vi "sv_Check for Midband Frequency Change.vi"(8 "error in (no error)":errorcluster, 10 "midband frequency setting":T1, 11 "reset filter (F)":bool) -> (0 "error out":errorcluster, 3 "parameter has changed":bool)   [LabVIEW 2017, in "SoundVib_Octave_2014 standard.lvlib"]
uses:
  <vilib>/addons/Sound and Vibration/svt_Octave/SoundVib_Octave_2014 standard.lvlib
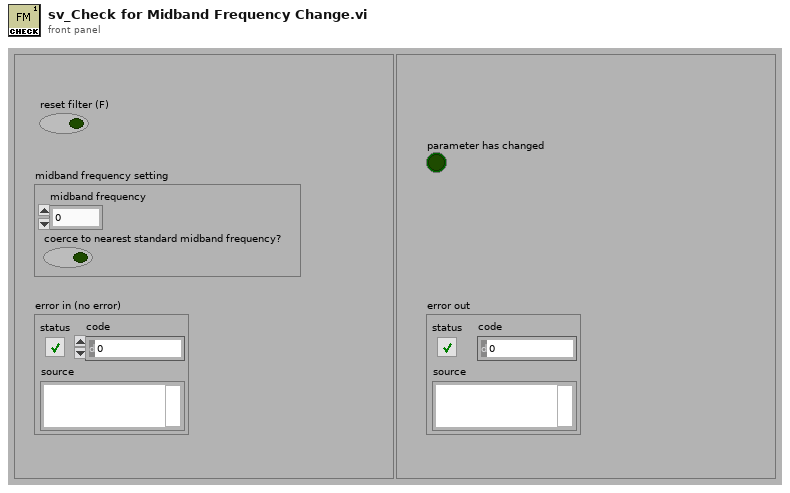
[diagram p1: front panel]
types:
  T1 = cluster{"midband frequency":dbl, "coerce to nearest standard midband frequency?":bool}
  T2 = cluster{"midband frequency":bool, "coerce to nearest standard midband frequency?":bool}
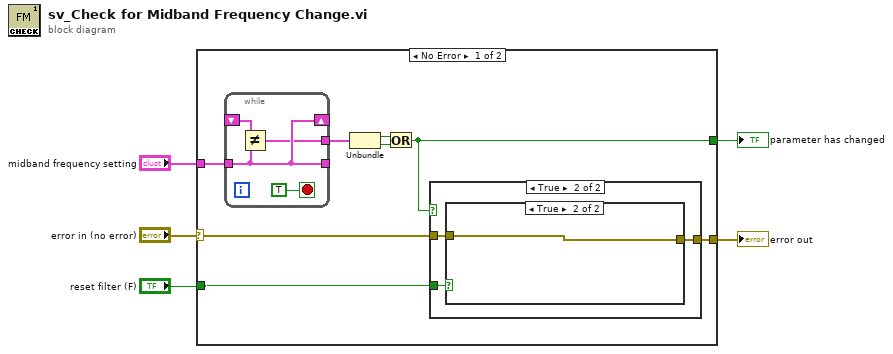
[diagram p0: block diagram]
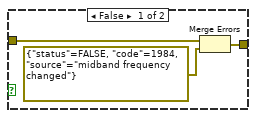
[diagram p3: hidden frame]
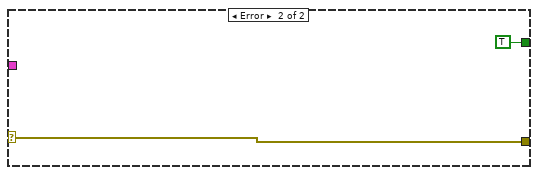
[diagram p4: hidden frame]
diagram:
  n1 = case shown="No Error" "error in (no error)" {
    selector: "error in (no error)" -> [w12 w27]
    tunnel: [w11 w27] -> w4
    tunnel: "midband frequency setting" -> [w13 _]
    tunnel: [w6 TRUE] -> w3
    tunnel: "reset filter (F)" -> [w10 _]
    frame No Error {
      n2 = while {
        tunnel: [w15] -> _
        tunnel: w13 -> [w15]
        shift-left: _ -> [w16]
        shift-right: [w15] -> _
        tunnel: [w14] -> w9
        stop <- TRUE stop-if-true
        n3 = Not Equal?(x=w16, y=w15) -> (x != y?=w14:T2)
      }
      n4 = Unbundle(w9) -> ("midband frequency"=w8:bool, "coerce to nearest standard midband frequency?"=w7:bool)
      n5 = Or(x=w8, y=w7) -> (x .or. y?=w6:bool)
      n6 = case shown="True" w6 {
        tunnel: w12 -> [w18 w19]
        tunnel: [w18 w21] -> w11
        tunnel: w10 -> [_ w20]
        frame False {
        }
        frame True {
          n7 = case shown="True" w20 {
            tunnel: [w23 w25] -> w21
            tunnel: w19 -> [w22 w25]
            frame False {
              n8 = Merge Errors(w22, errorcluster {"status"=FALSE, "code"=1984, "source"="midband frequency changed"} ("error IO")) -> (w23:errorcluster)
            }
            frame True {
            }
          }
        }
      }
    }
    frame Error {
    }
  }
  "error out" <- w4
  "parameter has changed" <- w3
